vi "init runtime test.vi"() -> ()   [LabVIEW 2013, in "sample module tests.lvlib"]
uses:
  sample module tests.lvlib
  module/execution/sample module runtime.lvclass
  <vilib>/NI/Tag Bus/tag/tag descriptor.lvclass/tag descriptor.ctl
  channel/TBM channel.lvclass/TBM channel.ctl
  <vilib>/NI/Tag Bus/tag/read tag name.vi
  <vilib>/NI/Tag Bus/tag/read data type.vi
  channel/Read channel classification.vi
  channel/TBM channel.lvclass
  <vilib>/NI/Tag Bus/dictionary/data dictionary.lvclass
panel:
  out "tags found":bool
  out "no error":errorcluster
  out "expected execution settings":bool
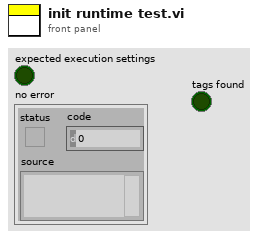
[diagram p1: front panel]
types:
  T1 = typedef "TBM channel.lvclass/data tables.ctl" = cluster{"input data":T2, "processing parameter":T2, "processing result":T2, "output data":T2}
  T2 = typedef "tag bus.lvlib/dictionary table pair.ctl" = cluster{"data dictionary":refnum<class "data dictionary.lvclass">, "data table":T3}
  T3 = typedef "tag bus.lvlib/data table.lvlib/data table.ctl" = cluster{"Double":dbl[], "Single":sgl[], "I64":i64[], "I32":i32[], "I16":i16[], "I8":i8[], "U64":u64[], "U32":u32[], "U16":u16[], "U8":u8[], "Boolean":bool[], "String":string[], "Array of Double":cluster{"DBL Array":dbl[]}[], "Array of Single":cluster{"SGL Array":sgl[]}[], "Array of I64":cluster{"I64 Array":i64[]}[], "Array of I32":cluster{"I32 Array":i32[]}[], "Array of I16":cluster{"I16 Array":i16[]}[], "Array of I8":cluster{"I8 Array":i8[]}[], "Array of U64":cluster{"U64 Array":u64[]}[], "Array of U32":cluster{"U32 Array":u32[]}[], "Array of U16":cluster{"U16 Array":u16[]}[], "Array of U8":cluster{"U8 Array":u8[]}[], "Array of Boolean":cluster{"Boolean Array":bool[]}[], "Array of String":cluster{"String Array":string[]}[]}
  T4 = typedef "TBM module execution interface.lvclass/execution settings.ctl" = cluster{"reads inputs":bool, "processes data":bool, "writes outputs":bool}
  T5 = typedef "tag bus.lvlib/tag descriptor.lvclass/Data Type.ctl" = enum16{"Double", "Single", "I64", "I32", "I16", "I8", "U64", "U32", "U16", "U8", "Boolean", "String", "Array of Double", "Array of Single", "Array of I64", "Array of I32", "Array of I16", "Array of I8", "Array of U64", "Array of U32", "Array of U16", "Array of U8", "Array of Boolean", "Array of String"}
  T6 = typedef "TBM channel.lvclass/channel classification.ctl" = enum16{"input data", "output data", "processing parameter", "processing result"}
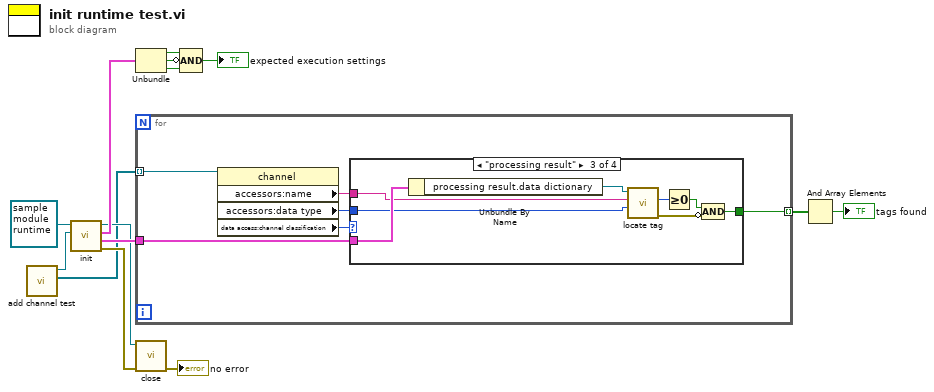
[diagram p0: block diagram]
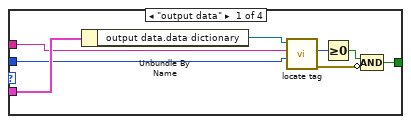
[diagram p2: hidden frame]
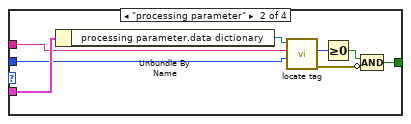
[diagram p3: hidden frame]
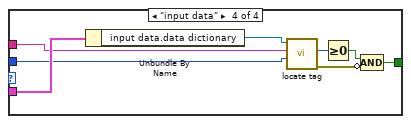
[diagram p4: hidden frame]
diagram:
  n1 = call "add channel test.vi"() -> ("channels"=w1:refnum<class "TBM channel.lvclass">[], "sample module configuration out"=w2:refnum<class "sample module configuration.lvclass">)  [unwired: 8 in, 2 out]
  n2 = call-dynamic "init.vi"("module configuration"=w2, "module in"=refnum<class "sample module runtime.lvclass"> refnum ("sample module")) -> ("error out"=w5:errorcluster, "data allocations"=w13:T1, "execution settings"=w12:T4, "module out"=w4:refnum<class "sample module runtime.lvclass">)  [unwired: 6 in]
  n3 = Unbundle(w12) -> ("reads inputs"=w11:bool, "processes data"=w9:bool, "writes outputs"=w10:bool)
  n4 = for {
    tunnel: w13 -> [w20]
    tunnel: w1 -> [w19] mode=indexing
    tunnel: [w18] -> w7 mode=indexing
    n5 = property class="channel"(reference=w19) -> ("accessors:name"=w15:string, "accessors:data type"=w16:T5, "data access:channel classification"=w17:T6)  [unwired: 1 in, 2 out]
    n6 = case shown="\"processing result\"" w17 {
      tunnel: w20 -> [w28 w36 w44 w52]
      tunnel: w16 -> [w26 w34 w42 w50]
      tunnel: w15 -> [w25 w33 w41 w49]
      tunnel: [w21 w29 w37 w45] -> w18
      frame "output data" {
        n7 = Unbundle By Name(w28) -> ("output data.data dictionary"=w27:refnum<class "data dictionary.lvclass">)
        n8 = call <vilib>:"locate tag.vi"("data type"=w26, "name"=w25, "data dictionary in"=w27) -> ("error out"=w22:errorcluster, "index"=w24:i32)  [unwired: 6 in, 1 out]
        n9 = Greater Or Equal To 0?(x=w24) -> (x >= 0?=w23:bool)
        n10 = Compound Arithmetic op=AND(w23, invert w22) -> (w21:bool)
      }
      frame "processing parameter" {
        n11 = Unbundle By Name(w36) -> ("processing parameter.data dictionary"=w35:refnum<class "data dictionary.lvclass">)
        n12 = call <vilib>:"locate tag.vi"("data type"=w34, "name"=w33, "data dictionary in"=w35) -> ("error out"=w30:errorcluster, "index"=w32:i32)  [unwired: 6 in, 1 out]
        n13 = Greater Or Equal To 0?(x=w32) -> (x >= 0?=w31:bool)
        n14 = Compound Arithmetic op=AND(w31, invert w30) -> (w29:bool)
      }
      frame "processing result" {
        n15 = Unbundle By Name(w44) -> ("processing result.data dictionary"=w43:refnum<class "data dictionary.lvclass">)
        n16 = call <vilib>:"locate tag.vi"("data type"=w42, "name"=w41, "data dictionary in"=w43) -> ("error out"=w38:errorcluster, "index"=w40:i32)  [unwired: 6 in, 1 out]
        n17 = Greater Or Equal To 0?(x=w40) -> (x >= 0?=w39:bool)
        n18 = Compound Arithmetic op=AND(w39, invert w38) -> (w37:bool)
      }
      frame "input data" {
        n19 = Unbundle By Name(w52) -> ("input data.data dictionary"=w51:refnum<class "data dictionary.lvclass">)
        n20 = call <vilib>:"locate tag.vi"("data type"=w50, "name"=w49, "data dictionary in"=w51) -> ("error out"=w46:errorcluster, "index"=w48:i32)  [unwired: 6 in, 1 out]
        n21 = Greater Or Equal To 0?(x=w48) -> (x >= 0?=w47:bool)
        n22 = Compound Arithmetic op=AND(w47, invert w46) -> (w45:bool)
      }
    }
  }
  n23 = call-dynamic "close.vi"("error in"=w5, "module in"=w4) -> ("error out"=→"no error":errorcluster)  [unwired: 9 in]
  n24 = Compound Arithmetic op=AND(w11, invert w9, w10) -> (→"expected execution settings":bool)
  n25 = And Array Elements(Boolean array=w7) -> (logical AND=→"tags found":bool)
